vi "PH_gentec_Powermeter.set Zero.vi"(0 "i ref in":refnum<vi>, 2 "VISA resource in":refnum<visa-resource-name>, 4 "Device error in":errorcluster, 5 "error in":errorcluster) -> (14 "i ref out":refnum<vi>, 15 "Timeout":bool, 16 "VISA resource out":refnum<visa-resource-name>, 17 "Error Message":string, 18 "Device error out":errorcluster, 19 "error out":errorcluster)   [LabVIEW 2014, in "PH_gentec_Powermeter.lvlib"]
doc: "This VI zeros the powermeter."
uses:
  PH_gentec_Powermeter.lvlib
  instr.lib/gentec-SOLO-PE/Driver/Type Defs/gentec-SOLO-PE.Zero Offset.ctl
  instr.lib/gentec-SOLO-PE/gentec-SOLO-PE - Driver.lvlib
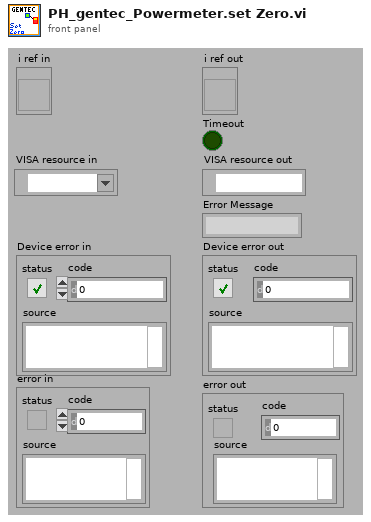
[diagram p1: front panel]
types:
  T1 = typedef "PH_gentec_Powermeter.lvlib/PH_gentec_Powermeter.i attribute.ctl" = cluster{"GUI References":cluster{"delete":refnum<vi>, "start stop Statistics":refnum<vi>, "Statistic Data":refnum<vi>, "Configuration Values":refnum<vi>, "Set Zero":refnum<vi>, "Data Sampling Settings":refnum<vi>, "Wanted Sets":refnum<vi>, "Current Sets":refnum<vi>}, "Start Stop Statistics":bool, "Wanted Sets":T2, "Current Sets":T2}
  T2 = typedef "PH_gentec_Powermeter.lvlib/PH_gentec_Powermeter.Sets.ctl" = cluster{"Data Sampling Settings":T3, "Set Zero":bool}
  T3 = typedef "gentec-SOLO-PE - Driver.lvlib/gentec-SOLO-PE.Data Sampling Settings.ctl" = cluster{"Sample Rate":u32, "Sample Rate Unit":u32, "Sample Period":u32, "Sample Period Unit":u32, "Total Duration":u32, "Total Duration Unit":u32, "Time Stamp":u32}
  T4 = typedef "gentec-SOLO-PE - Driver.lvlib/gentec-SOLO-PE.Zero Offset.ctl" = u32
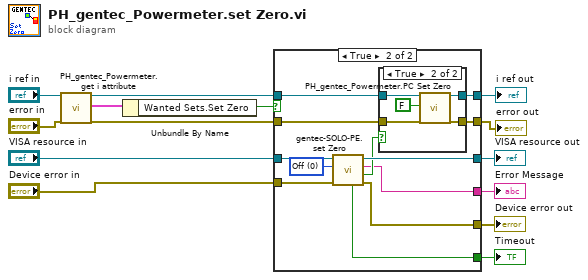
[diagram p0: block diagram]
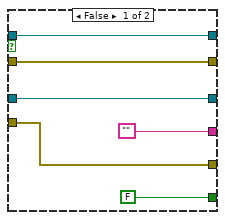
[diagram p2: hidden frame]
diagram:
  n1 = call "PH_gentec_Powermeter.get i attribute.vi"("i ref in"="i ref in", "error in (no error)"="error in") -> ("i ref out"=w8:refnum<vi>, "i attribute"=w10:T1, "error out"=w7:errorcluster)  [unwired: 15 in]
  n2 = Unbundle By Name(w10) -> ("Wanted Sets.Set Zero"=w3:bool)
  n3 = case shown="True" w3 {
    tunnel: [w20 w30] -> w14
    tunnel: [w19 w29] -> w12
    tunnel: "VISA resource in" -> [w18 w28]
    tunnel: w8 -> [w20 w32]
    tunnel: w7 -> [w19 w31]
    tunnel: [w18 w25] -> w6
    tunnel: [w17 w24] -> w5
    tunnel: "Device error in" -> [w17 w27]
    tunnel: ["" w22] -> w1
    tunnel: [FALSE ("Timeout") w21] -> w2
    frame False {
    }
    frame True {
      w26 = T4 0 items=["Off", "ReZero", "Undo"] ("Operation")
      n4 = call "gentec-SOLO-PE.set Zero.vi"("error in (no error)"=w27, "Zero Offset Operation"=w26, "VISA Refnum in"=w28) -> ("error out"=w24:errorcluster, "Acknoledged?"=w23:bool, "Error"=w22:string, "VISA Refnum out"=w25:refnum<visa-resource-name>, "Timeout"=w21:bool)  [unwired: 4 in]
      n5 = case shown="True" w23 {
        tunnel: w32 -> [w34 w39]
        tunnel: w31 -> [w33 w38]
        tunnel: [w34 w37] -> w30
        tunnel: [w33 w36] -> w29
        frame False {
        }
        frame True {
          n6 = call "PH_gentec_Powermeter.PC Set Zero.vi"("VI in"=w39, "Set Zero"=FALSE, "error in (no error)"=w38) -> ("VI out"=w37:refnum<vi>, "error out"=w36:errorcluster)  [unwired: 15 in]
        }
      }
    }
  }
  "error out" <- w12
  "i ref out" <- w14
  "VISA resource out" <- w6
  "Device error out" <- w5
  "Timeout" <- w2
  "Error Message" <- w1
